vi "test_basic.vi"() -> ()   [LabVIEW 2016]
panel:
  in  "System locator":string(combo)="usb:id:425839965"
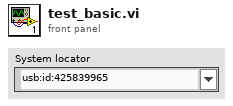
[diagram p1: front panel]
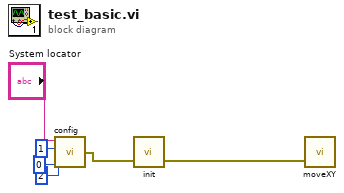
[diagram p0: block diagram]
diagram:
  n1 = call "config.vi"("System locator"="System locator", "X channel"=u32 1, "Y channel"=u32 2, "Rotation channel"=u32 0) -> ("error out"=w1:errorcluster)  [unwired: 1 in]
  n2 = call "init.vi"("error in (no error)"=w1) -> ("error out"=w3:errorcluster)  [unwired: 2 in]
  n3 = call "moveXY.vi"("error in (no error)"=w3) -> ()  [unwired: 2 in, 1 out]
